vi "AMM_Install Script.vi"(8 "error in (no error)":errorcluster) -> (0 "error out":errorcluster)   [LabVIEW 2014]
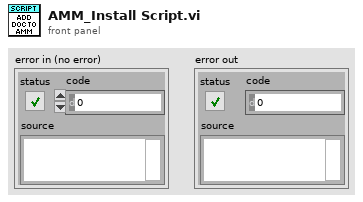
[diagram p1: front panel]
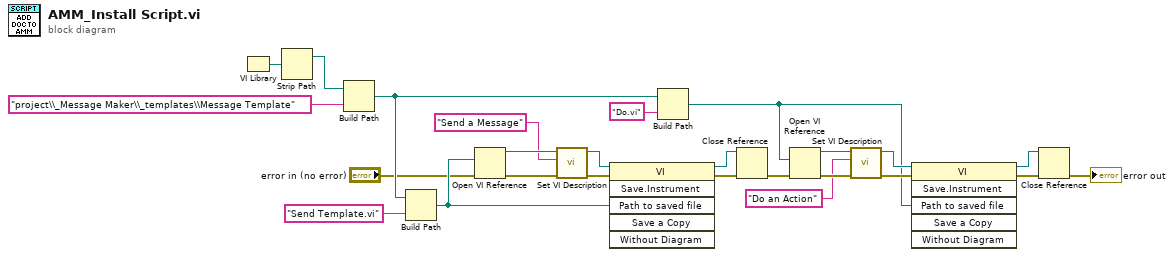
[diagram p0: block diagram]
diagram:
  n1 = VI Library() -> (path=w22:path)
  n2 = Strip Path(path=w22) -> (stripped path=w23:path)  [unwired: 1 out]
  n3 = Build Path(base path=w23, name or relative path="project\\_Message Maker\\_templates\\Message Template") -> (appended path=w20:path)
  n4 = Build Path(base path=w20, name or relative path="Send Template.vi") -> (appended path=w11:path)
  n5 = Open VI Reference(vi path=w11, error in (no error)="error in (no error)") -> (vi reference=w19:refnum<vi>, error out=w18:errorcluster)  [unwired: 4 in]
  n6 = call "Set VI Description.vi"("error in (no error)"=w18, "VI Description"="Send a Message", "VI"=w19) -> ("error out"=w12:errorcluster, "VI out"=w13:refnum<vi>)  [unwired: 7 in]
  n7 = invoke class="VI" method="Save.Instrument"(reference=w13, error in=w12, "Path to saved file"=w11) -> (reference out=w4:refnum<vi>, error out=w5:errorcluster)  [unwired: 3 in, 4 out]
  n8 = Build Path(base path=w20, name or relative path="Do.vi") -> (appended path=w8:path)
  n9 = Close Reference(reference=w4, error in (no error)=w5) -> (error out=w3:errorcluster)
  n10 = Open VI Reference(vi path=w8, error in (no error)=w3) -> (vi reference=w16:refnum<vi>, error out=w17:errorcluster)  [unwired: 4 in]
  n11 = call "Set VI Description.vi"("error in (no error)"=w17, "VI Description"="Do an Action", "VI"=w16) -> ("error out"=w9:errorcluster, "VI out"=w10:refnum<vi>)  [unwired: 7 in]
  n12 = invoke class="VI" method="Save.Instrument"(reference=w10, error in=w9, "Path to saved file"=w8) -> (reference out=w6:refnum<vi>, error out=w7:errorcluster)  [unwired: 3 in, 4 out]
  n13 = Close Reference(reference=w6, error in (no error)=w7) -> (error out=→"error out":errorcluster)
